vi "Teleop Actions.vi"   [LabVIEW 2018]
uses:
  <vilib>/Rock Robotics/WPI/Solenoid/WPI_SolenoidValue.ctl
  Framework/Robot Global Data.vi
types:
  T1 = typedef "Command Status Info.ctl" = cluster{"Name":string, "Status":T2, "notifier out":T3}
  T2 = typedef "Completion Status.ctl" = enum16{"Successful", "Aborted", "Incomplete"}
  T3 = typedef "Completion Notifier.ctl" = refnum<notifier>
  T4 = typedef "WPI_SolenoidValue.ctl" = enum16{"Off", "On", "Forward", "Reverse"}
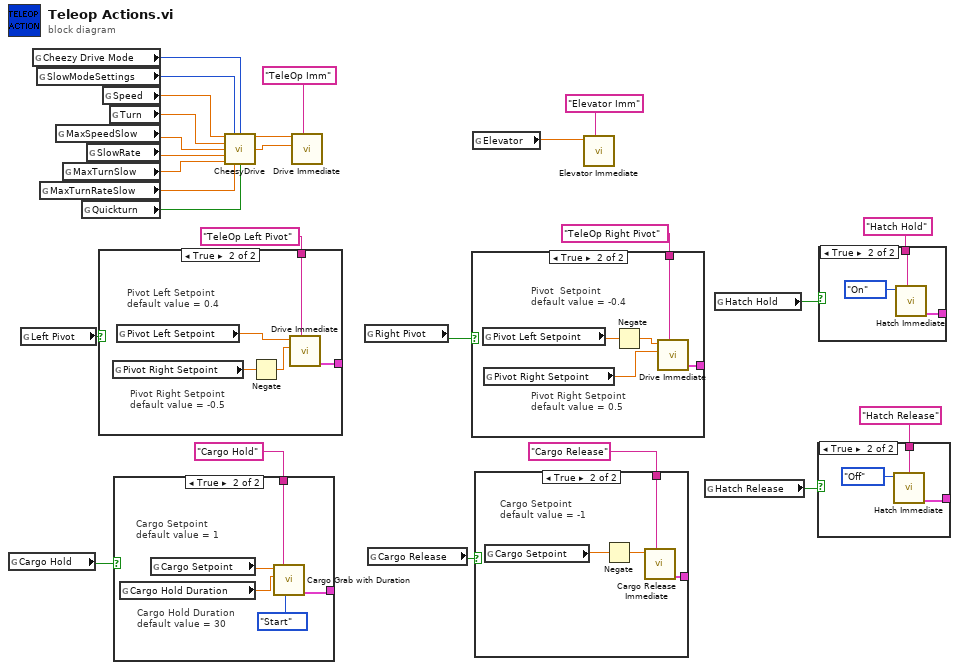
[diagram p0: block diagram]
diagram:
  n1 = global read "Robot Global Data.vi" "Cargo Hold"() -> (w6:bool)
  n2 = global read "Robot Global Data.vi" "Left Pivot"() -> (w22:bool)
  n3 = global read "Robot Global Data.vi" "Cheezy Drive Mode"() -> (w21:u32)
  n4 = global read "Robot Global Data.vi" "SlowModeSettings"() -> (w11:i32)
  n5 = global read "Robot Global Data.vi" "MaxTurnRateSlow"() -> (w13:dbl)
  n6 = global read "Robot Global Data.vi" "MaxSpeedSlow"() -> (w16:dbl)
  n7 = global read "Robot Global Data.vi" "MaxTurnSlow"() -> (w14:dbl)
  n8 = global read "Robot Global Data.vi" "Quickturn"() -> (w12:bool)
  n9 = global read "Robot Global Data.vi" "SlowRate"() -> (w15:dbl)
  n10 = case shown="True" w22 {
    tunnel: [_ w31] -> _
    tunnel: "TeleOp Left Pivot" ("Description") -> [_ w30]
    frame False {
    }
    frame True {
      # "Pivot Right Setpoint\ndefault value = -0.5"
      # "Pivot Left Setpoint\ndefault value = 0.4"
      n11 = global read "Robot Global Data.vi" "Pivot Right Setpoint"() -> (w28:dbl)
      n12 = global read "Robot Global Data.vi" "Pivot Left Setpoint"() -> (w29:dbl)
      n13 = Negate(x=w28) -> (-x=w27:dbl)
      n14 = call "Drive Immediate.vi"("Description"=w30, "Right Setpoint"=w27, "Left Setpoint"=w29) -> ("Command Info Out"=w31:T1)  [unwired: 8 in]
    }
  }
  n15 = global read "Robot Global Data.vi" "Speed"() -> (w18:dbl)
  n16 = global read "Robot Global Data.vi" "Turn"() -> (w17:dbl)
  n17 = case shown="True" w6 {
    tunnel: [_ w36] -> _
    tunnel: "Cargo Hold" ("Description") -> [_ w35]
    frame False {
    }
    frame True {
      # "Cargo Hold Duration\ndefault value = 30"
      # "Cargo Setpoint\ndefault value = 1"
      n18 = global read "Robot Global Data.vi" "Cargo Hold Duration"() -> (w32:dbl)
      n19 = global read "Robot Global Data.vi" "Cargo Setpoint"() -> (w34:dbl)
      n20 = call "Cargo Grab with Duration.vi"("Synchronization"=enum16{"Start", "Wait"}."Start", "Description"=w35, "Duration (s)"=w32, "Setpoint"=w34) -> ("Command Info Out"=w36:T1)  [unwired: 7 in]
    }
  }
  n21 = call "CheesyDrive.vi"("Throttle"=w18, "SlowModeSettings"=w11, "SlowMode"=w21, "Wheel"=w17, "MaxSpeedSlow"=w16, "SlowRate"=w15, "MaxTurnSlow"=w14, "MaxTurnRateSlow"=w13, "Quickturn"=w12) -> ("Left PWM"=w20:dbl, "Right PWM"=w19:dbl)  [unwired: 5 in]
  n22 = call "Drive Immediate.vi"("Description"="TeleOp Imm", "Right Setpoint"=w19, "Left Setpoint"=w20) -> ()  [unwired: 8 in, 1 out]
  n23 = global read "Robot Global Data.vi" "Right Pivot"() -> (w23:bool)
  n24 = global read "Robot Global Data.vi" "Cargo Release"() -> (w5:bool)
  n25 = case shown="True" w23 {
    tunnel: [_ w41] -> _
    tunnel: "TeleOp Right Pivot" ("Description") -> [_ w40]
    frame False {
    }
    frame True {
      # "Pivot Right Setpoint\ndefault value = 0.5"
      # "Pivot  Setpoint\ndefault value = -0.4"
      n26 = global read "Robot Global Data.vi" "Pivot Left Setpoint"() -> (w38:dbl)
      n27 = global read "Robot Global Data.vi" "Pivot Right Setpoint"() -> (w39:dbl)
      n28 = Negate(x=w38) -> (-x=w37:dbl)
      n29 = call "Drive Immediate.vi"("Description"=w40, "Right Setpoint"=w39, "Left Setpoint"=w37) -> ("Command Info Out"=w41:T1)  [unwired: 8 in]
    }
  }
  n30 = global read "Robot Global Data.vi" "Elevator"() -> (w10:dbl)
  n31 = case shown="True" w5 {
    tunnel: [_ w45] -> _
    tunnel: "Cargo Release" ("Description") -> [_ w44]
    frame False {
    }
    frame True {
      # "Cargo Setpoint\ndefault value = -1"
      n32 = global read "Robot Global Data.vi" "Cargo Setpoint"() -> (w43:dbl)
      n33 = Negate(x=w43) -> (-x=w42:dbl)
      n34 = call "Cargo Release Immediate.vi"("Description"=w44, "Setpoint"=w42) -> ("Command Info Out"=w45:T1)  [unwired: 9 in]
    }
  }
  n35 = call "Elevator Immediate.vi"("Description"="Elevator Imm", "Setpoint"=w10) -> ()  [unwired: 9 in, 1 out]
  n36 = global read "Robot Global Data.vi" "Hatch Release"() -> (w2:bool)
  n37 = global read "Robot Global Data.vi" "Hatch Hold"() -> (w1:bool)
  n38 = case shown="True" w2 {
    tunnel: "Hatch Release" ("Description") -> [_ w48]
    tunnel: [_ w47] -> _
    frame False {
    }
    frame True {
      n39 = call "Hatch Immediate.vi"("Description"=w48, "Relay Value"=WPI_SolenoidValue."Off" ("Hatch Action")) -> ("Command Info Out"=w47:T1)  [unwired: 9 in]
    }
  }
  n40 = case shown="True" w1 {
    tunnel: "Hatch Hold" ("Description") -> [_ w51]
    tunnel: [_ w50] -> _
    frame False {
    }
    frame True {
      n41 = call "Hatch Immediate.vi"("Description"=w51, "Relay Value"=WPI_SolenoidValue."On" ("Hatch Action")) -> ("Command Info Out"=w50:T1)  [unwired: 9 in]
    }
  }
